vi "MAX31855.vi"() -> (7 "Temperatura giunzione 2":fxp<+,17,12>)   [LabVIEW 2012]
uses:
  <vilib>/rvi/eio/common/nirviEmuTemplateMethod_errors.vi
  <vilib>/eio/EIONode/EIONode.xnode
panel:
  out "T OIL":u32
  out "T H2O":u32
  out "T FUEL":u32
  out "T AIR":u32
  out "Temperatura TC 2":fxp<+,17,14> format="%.8g"
  out "FAULT 2":bool=TRUE
  out "Short Circuit GND 2":bool=TRUE
  out "Open Circuit Fault 2":bool=TRUE
  out "Short Ciruit VCC 2":bool=TRUE
  out "Temperatura giunzione 1":fxp<+,17,12>
  out "Short Ciruit VCC 1":bool=TRUE
  out "Open Circuit Fault 1":bool=TRUE
  out "Short Circuit GND 1":bool=TRUE
  out "FAULT 1":bool=TRUE
  out "Temperatura TC 1":fxp<+,17,14> format="%.8g"
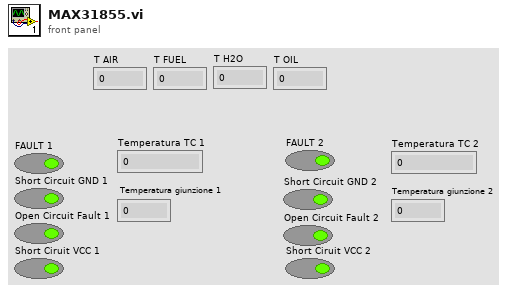
[diagram p1: front panel]
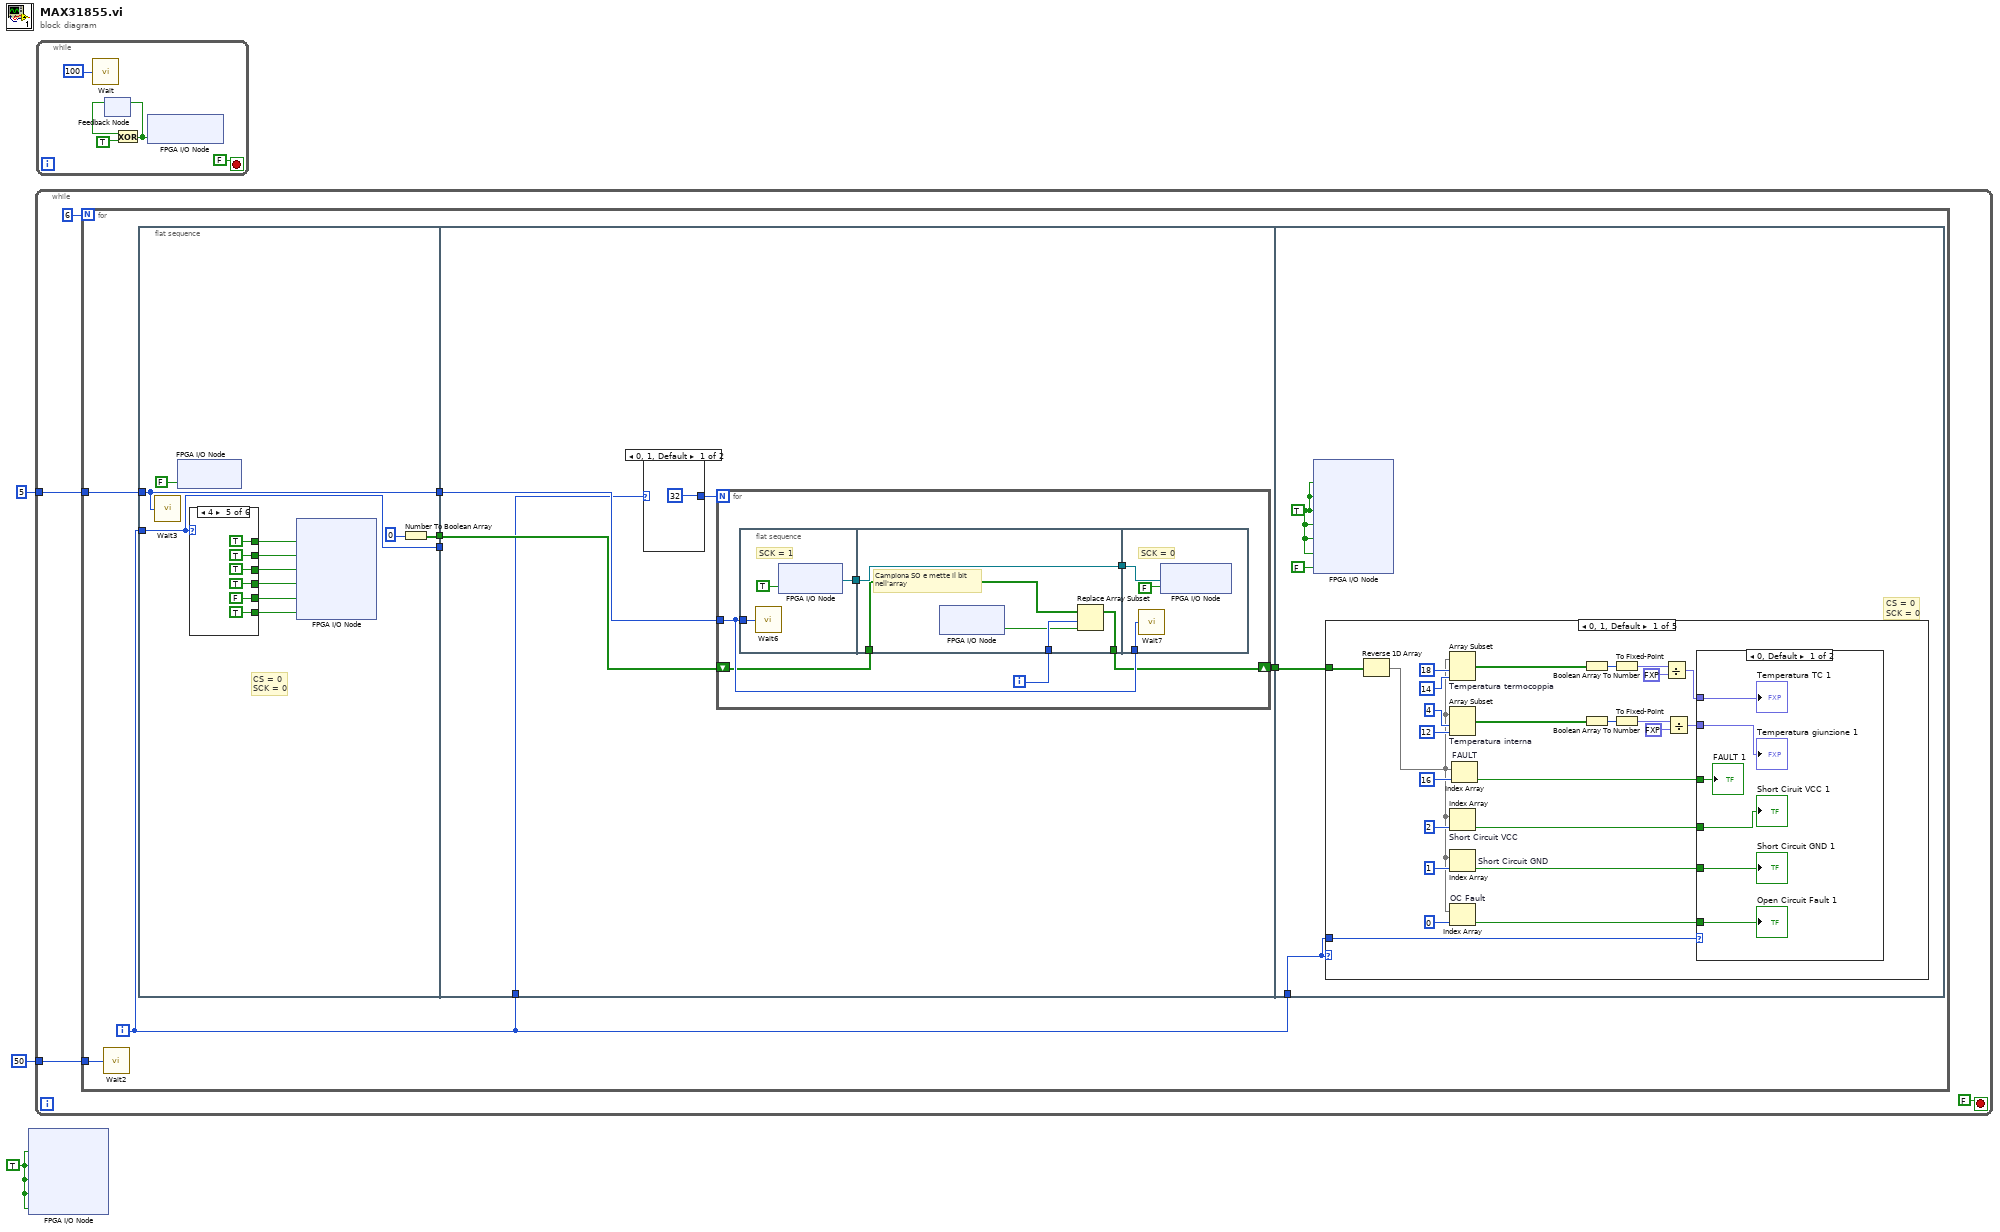
[diagram p0: block diagram]
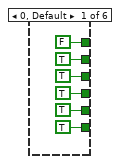
[diagram p2: hidden frame]
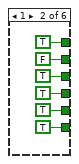
[diagram p3: hidden frame]
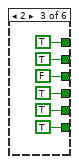
[diagram p4: hidden frame]
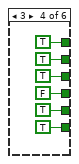
[diagram p5: hidden frame]
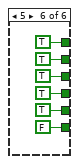
[diagram p6: hidden frame]
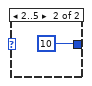
[diagram p7: hidden frame]
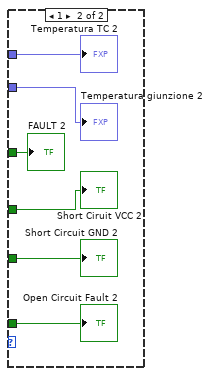
[diagram p8: hidden frame]
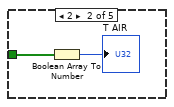
[diagram p9: hidden frame]
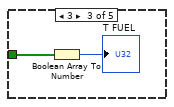
[diagram p10: hidden frame]
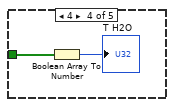
[diagram p11: hidden frame]
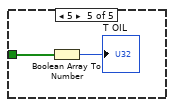
[diagram p12: hidden frame]
diagram:
  w1 = TRUE ("CS_TCK2#")
  n1 = xnode "FPGA I/O Node"("CS_TCK2#"=w1, "CSAIR"=w1, "CSFUEL"=w1, "CSH2O"=w1, "CSOIL"=w1) -> ()  [unwired: 5 in, 5 out]
  n2 = while {
    tunnel: u32 5 -> [w6]
    tunnel: u32 50 ("Count(mSec)") -> [w4]
    stop <- FALSE stop-if-true
    n3 = for {
      N: 6 -> [_]
      tunnel: w6 -> [w11]
      tunnel: w4 -> [w10]
      i -> [w8]
      n4 = call "Wait2"("Count(mSec)"=w10) -> ()  [unwired: 1 out]
      n5 = flat-sequence {
        tunnel: [w24] -> w14
        tunnel: w11 -> [w24]
        tunnel: [w22] -> w13
        tunnel: w8 -> [w19]
        tunnel: [w19] -> w9
        tunnel: [w66] -> w12
        tunnel: w14 -> [w65]
        tunnel: w13 -> [w64]
        tunnel: w9 -> [_]
        tunnel: w8 -> [w62]
        tunnel: w12 -> [w89]
        tunnel: w8 -> [w87]
        frame #0 {
          # "CS = 0\nSCK = 0"
          n6 = call "Wait3"("Count(uSec)"=w24) -> ()  [unwired: 1 out]
          n7 = xnode "FPGA I/O Node"("SCK"=FALSE ("RMC/DIO48")) -> ()  [unwired: 1 in, 1 out]
          n8 = case shown="4" w19 {
            tunnel: [FALSE TRUE ("CS_TCK1#") TRUE ("CS_TCK1#") TRUE ("CS_TCK1#") TRUE ("CS_TCK1#") TRUE ("CS_TCK1#")] -> w21
            tunnel: [TRUE FALSE TRUE TRUE TRUE TRUE] -> w20
            tunnel: [TRUE TRUE FALSE TRUE TRUE TRUE] -> w18
            tunnel: [TRUE TRUE TRUE FALSE TRUE TRUE] -> w17
            tunnel: [TRUE TRUE TRUE TRUE FALSE TRUE] -> w16
            tunnel: [TRUE TRUE TRUE TRUE TRUE FALSE] -> w15
            frame 0, Default {
            }
            frame 1 {
            }
            frame 2 {
            }
            frame 3 {
            }
            frame 4 {
            }
            frame 5 {
            }
          }
          n9 = xnode "FPGA I/O Node"("CS_TCK1#"=w21, "CS_TCK2#"=w20, "CSAIR"=w18, "CSFUEL"=w17, "CSH2O"=w16, "CSOIL"=w15) -> ()  [unwired: 6 in, 6 out]
          n10 = Number To Boolean Array(number=u32 0) -> (Boolean array=w22:bool[])
        }
        frame #1 {
          n11 = case shown="0, 1, Default" w62 {
            tunnel: [32 10] -> w63
            frame 0, 1, Default {
            }
            frame 2..5 {
            }
          }
          n12 = for {
            N: w63 -> [_]
            tunnel: w65 -> [w71]
            shift-right: [w70] -> w66
            shift-left: w64 -> [w69]
            i -> [w72]
            n13 = flat-sequence {
              tunnel: [w77] -> w73
              tunnel: w71 -> [w76]
              tunnel: [w82] -> w74
              tunnel: w73 -> [w82]
              tunnel: w72 -> [w81]
              tunnel: [w78] -> w70
              tunnel: w69 -> [w79]
              tunnel: w74 -> [w85]
              tunnel: w71 -> [w83]
              frame #0 {
                # "SCK = 1"
                n14 = call "Wait6"("Count(uSec)"=w76) -> ()  [unwired: 1 out]
                n15 = xnode "FPGA I/O Node"("SCK"=TRUE ("I/O Item")) -> ("FPGA I/O Out"=w77:refnum<k21>)  [unwired: 1 in]
              }
              frame #1 {
                # "Campiona SO e mette il bit\nnell'array"
                n16 = xnode "FPGA I/O Node"() -> ("SO"=w80:bool)  [unwired: 1 in, 1 out]
                n17 = Replace Array Subset(array=w79, new element=w80, index=w81) -> (w78:bool[])
              }
              frame #2 {
                # "SCK = 0"
                n18 = call "Wait7"("Count(uSec)"=w83) -> ()  [unwired: 1 out]
                n19 = xnode "FPGA I/O Node"("I/O Item"=FALSE, "FPGA I/O In"=w85) -> ()  [unwired: 1 out]
              }
            }
          }
        }
        frame #2 {
          w88 = TRUE ("I/O Item")
          # "CS = 0\nSCK = 0"
          n20 = xnode "FPGA I/O Node"("CSAIR"=w88, "CSFUEL"=w88, "CSH2O"=w88, "CSOIL"=w88, "CS_TCK1#"=w88, "CS_TCK2#"=w88, "SCK"=FALSE ("I/O Item")) -> ()  [unwired: 7 in, 7 out]
          n21 = case shown="0, 1, Default" w87 {
            tunnel: w89 -> [w104 w128 w130 w132 w134]
            tunnel: w87 -> [w90 _ _ _ _]
            frame 0, 1, Default {
              n22 = Reverse 1D Array(array=w104) -> (reversed array=w103:bool[])
              n23 = Array Subset "Temperatura termocoppia"(array=w103, index=18, length=14) -> (w112:bool[])
              n24 = Array Subset "Temperatura interna"(array=w103, index=4, length=12) -> (w111:bool[])
              n25 = Index Array "Short Circuit VCC"(array=w103, index=2) -> (element=w101:bool)
              n26 = Index Array "Short Circuit GND"(array=w103, index=1) -> (element=w100:bool)
              n27 = Index Array "OC Fault"(array=w103, index=0) -> (element=w99:bool)
              n28 = Index Array "FAULT"(array=w103, index=16) -> (element=w102:bool)
              n29 = Boolean Array To Number(Boolean array=w112) -> (number=w92:u16)
              n30 = Boolean Array To Number(Boolean array=w111) -> (number=w97:u16)
              n31 = To Fixed-Point(number=w92) -> (fixed-point=w93:fxp<+,16,16>)  [unwired: 1 in]
              n32 = To Fixed-Point(number=w97) -> (fixed-point=w96:fxp<+,16,16>)  [unwired: 1 in]
              n33 = Divide(x=w93, y=fxp<+,1,3> 4.0) -> (x/y=w91:fxp<+,17,14>)
              n34 = Divide(x=w96, y=fxp<+,1,5> 16.0) -> (x/y=w95:fxp<+,17,12>)
              n35 = case shown="0, Default" w90 {
                tunnel: w102 -> [w120 w126]
                tunnel: w101 -> [w119 w125]
                tunnel: w100 -> [w118 w124]
                tunnel: w99 -> [w117 w123]
                tunnel: w95 -> [w116 w122]
                tunnel: w91 -> [w115 w121]
                frame 0, Default {
                  "Temperatura TC 1" <- w115
                  "FAULT 1" <- w120
                  "Short Circuit GND 1" <- w118
                  "Open Circuit Fault 1" <- w117
                  "Short Ciruit VCC 1" <- w119
                  "Temperatura giunzione 1" <- w116
                }
                frame 1 {
                  "Temperatura TC 2" <- w121
                  "FAULT 2" <- w126
                  "Short Circuit GND 2" <- w124
                  "Open Circuit Fault 2" <- w123
                  "Short Ciruit VCC 2" <- w125
                  "Temperatura giunzione 2" <- w122
                }
              }
            }
            frame 2 {
              n36 = Boolean Array To Number(Boolean array=w128) -> (number=→"T AIR":u32)
            }
            frame 3 {
              n37 = Boolean Array To Number(Boolean array=w130) -> (number=→"T FUEL":u32)
            }
            frame 4 {
              n38 = Boolean Array To Number(Boolean array=w132) -> (number=→"T H2O":u32)
            }
            frame 5 {
              n39 = Boolean Array To Number(Boolean array=w134) -> (number=→"T OIL":u32)
            }
          }
        }
      }
    }
  }
  n40 = while {
    stop <- FALSE stop-if-true
    n41 = call "Wait"("Count(mSec)"=u32 100) -> ()  [unwired: 1 out]
    n42 = feedback #1() -> (w136:bool)  [unwired: 1 in]
    n43 = Exclusive Or(1:TRUE ("y"), 2:w136) -> (0:w137:bool)
    n44 = feedback-in #1(w137) -> ()
    n45 = xnode "FPGA I/O Node"("FPGA LED"=w137) -> ()  [unwired: 1 in, 1 out]
  }
